vi "Command Channel Names DAO.vi"(7 "Config Ref  In":T1, 8 "error in (no error)":errorcluster, 9 "Names In":T2, 10 "LBCB Number":T3, 11 "Actions":T4) -> (0 "error out":errorcluster, 1 "Names Out":T2, 4 "Config Ref Out":T1)   [LabVIEW 2009]
uses:
  Metadata/Persistant DAO Actions.ctl
  Metadata/Actuator Channel Names.ctl
  Metadata/LBCB Number.ctl
  <vilib>/Utility/config.llb/Config Data RefNum.ctl
  <vilib>/Utility/config.llb/NI_LVConfig.lvlib
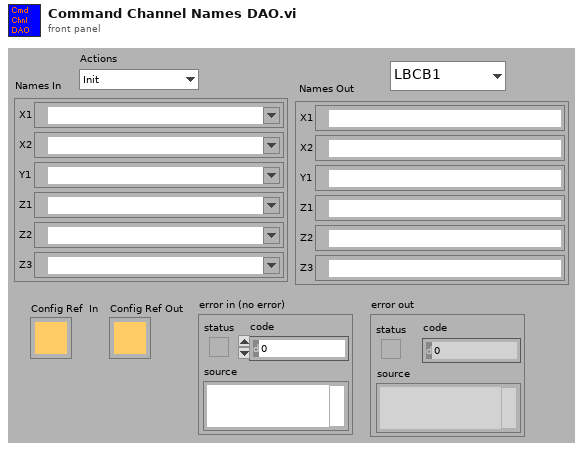
[diagram p1: front panel]
types:
  T1 = typedef "NI_LVConfig.lvlib/Config Data RefNum.ctl" = refnum<k1>
  T2 = typedef "Actuator Channel Names.ctl" = cluster{"X1":refnum<k21>, "X2":refnum<k21>, "Y1":refnum<k21>, "Z1":refnum<k21>, "Z2":refnum<k21>, "Z3":refnum<k21>}
  T3 = typedef "LBCB Number.ctl" = enum16{"LBCB1", "LBCB2"}
  T4 = typedef "Persistant DAO Actions.ctl" = enum16{"Init", "Get", "Set", "Load", "Save"}
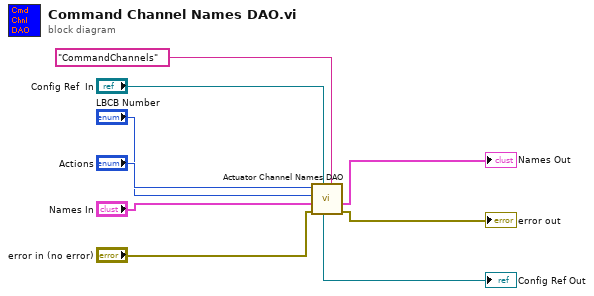
[diagram p0: block diagram]
diagram:
  n1 = call "Actuator Channel Names DAO.vi"("section"="CommandChannels", "Config Ref  In"="Config Ref  In", "error in (no error)"="error in (no error)", "Names In"="Names In", "LBCB Number"="LBCB Number", "Actions"="Actions") -> ("error out"=→"error out":errorcluster, "Names Out"=→"Names Out":T2, "Config Ref Out"=→"Config Ref Out":T1)  [unwired: 3 out]
